vi "UDPsender.vi"() -> ()   [LabVIEW 2012]
panel:
  in  "Relative Time Step":u32
  in  "Time Reset":bool
  in  "Harvest Mode":bool[](array[boolean])
  in  "Throttle Mode":u16
  in  "Test Modes":bool[](array[boolean])
  in  "Channel Test Mode Config":bool[](array[boolean])
  in  "Sync Test Mode Config":bool[](array[boolean])
  in  "Sync Select":bool[](array[boolean])
  in  "Profiles Per Histogram":u16
  in  "Number of Bins":u16
  in  "User Reset":bool
  in  "Counts Per Bin":u16
  in  "Reset Profile Accumulator":bool[](array[boolean])
  in  "Channel Enable":bool[](array[boolean])
  in  "Sync Enable":bool[](array[boolean])
  in  "Reset":bool
  in  "Send":bool
  in  "Send Command, manual entry":string
  out "Sender Error":errorcluster
  in  "End Sender Program":bool
  # "valid range (2-4096)"
  # "valid range (2-4096)"
  # "valid range (1-32,768)"
  # "stop sender"
  # "valid range (0-7)"
  # "valid range (0-33,554,432)"
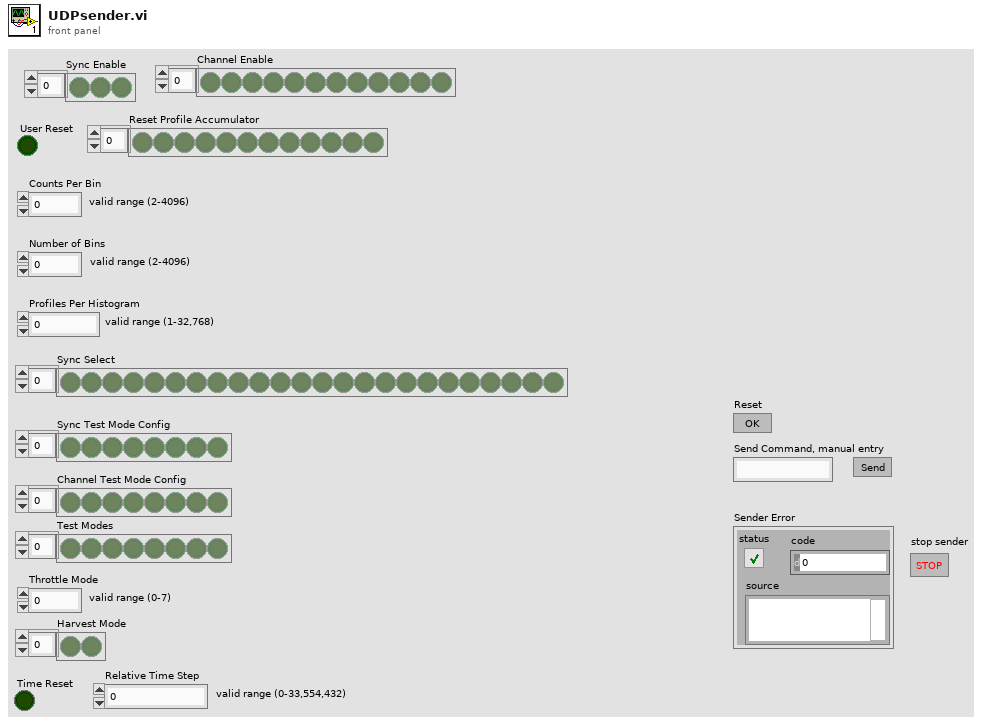
[diagram p1: front panel]
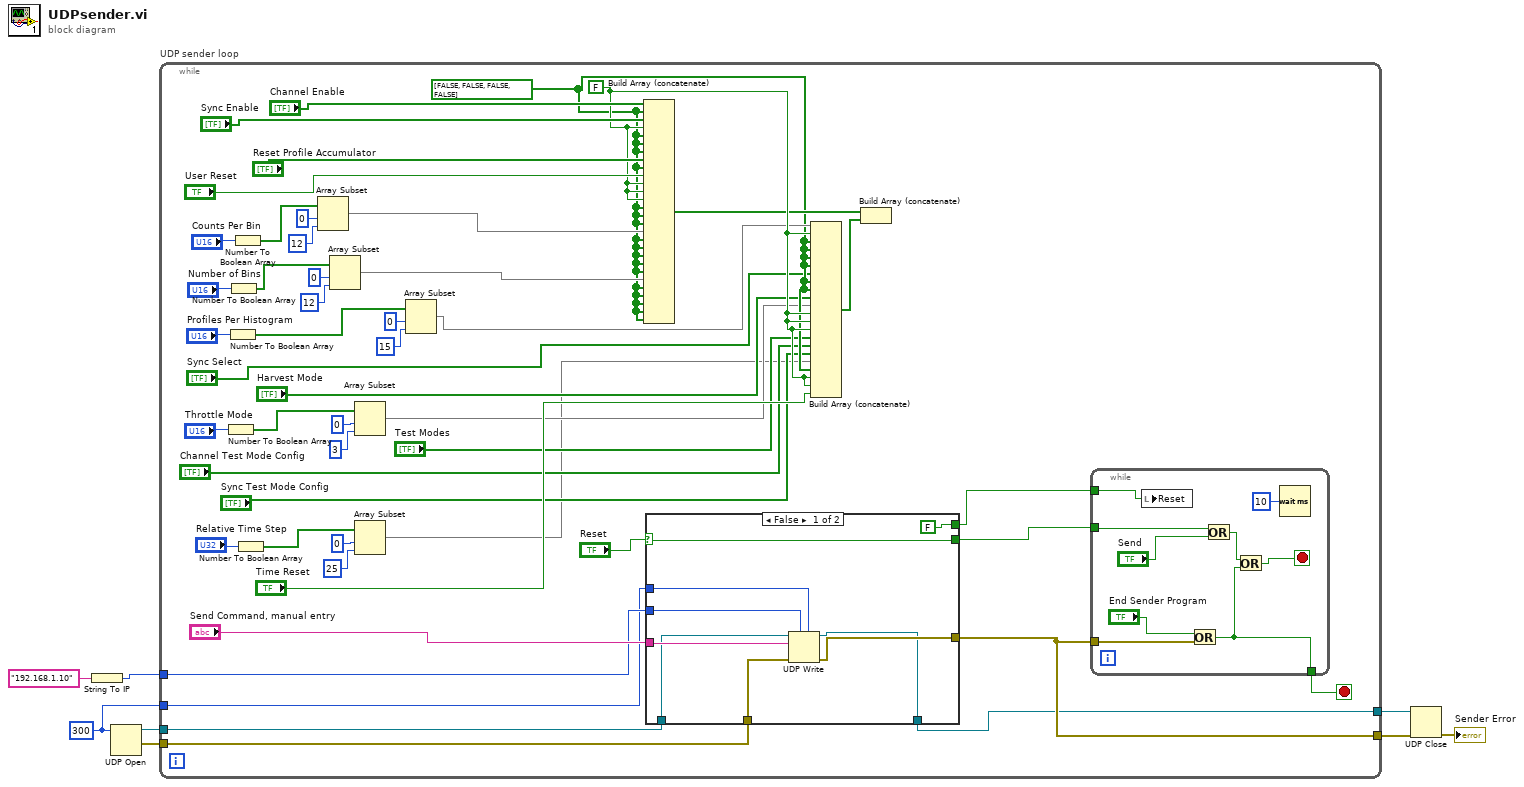
[diagram p0: block diagram]
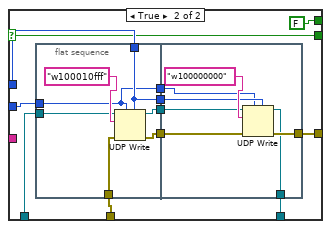
[diagram p2: hidden frame]
diagram:
  w1 = u16 300 ("port")
  n1 = String To IP(1:"192.168.1.10" ("name")) -> (0:w3:u32)
  n2 = UDP Open(11:w1) -> (port=w7:refnum<k16>, 0:w8:errorcluster)  [unwired: 4 in, 1 out]
  n3 = while "UDP sender loop" {
    tunnel: w8 -> [w55]
    tunnel: w7 -> [w53]
    tunnel: [w54] -> w6
    tunnel: w3 -> [w52]
    tunnel: [w25] -> w2
    tunnel: w1 -> [w50]
    stop <- w58 stop-if-true
    w16 = bool[] [FALSE, FALSE, FALSE, FALSE] ("appended array")
    w21 = FALSE ("Reset")
    n4 = Number To Boolean Array(number="Throttle Mode") -> (Boolean array=w26:bool[])
    n5 = Number To Boolean Array(number="Profiles Per Histogram") -> (Boolean array=w34:bool[])
    n6 = Number To Boolean Array(number="Number of Bins") -> (Boolean array=w37:bool[])
    n7 = Number To Boolean Array(number="Counts Per Bin") -> (Boolean array=w40:bool[])
    n8 = Number To Boolean Array(number="Relative Time Step") -> (Boolean array=w22:bool[])
    n9 = Array Subset(array=w40, index=0, length=12) -> (w30:bool[])
    n10 = Array Subset(array=w37, index=0, length=12) -> (w29:bool[])
    n11 = Array Subset(array=w26, index=0, length=3) -> (w13:bool[])
    n12 = Array Subset(array=w22, index=0, length=25) -> (w9:bool[])
    n13 = Array Subset(array=w34, index=0, length=15) -> (w17:bool[])
    n14 = Build Array (concatenate)("Channel Enable", w16, "Sync Enable", w21, w16, w16, w16, "Reset Profile Accumulator", w16, "User Reset", w21, w21, w21, w16, w16, w16, w30, w16, w16, w16, w16, w16, w29, w16, w16, w16, w16, w16) -> (w19:bool[])
    n15 = case shown="False" "Reset" {
      selector: "Reset" -> [w59 w68]
      tunnel: "Send Command, manual entry" -> [w67 _]
      tunnel: w55 -> [w65 w79]
      tunnel: [w64 w77] -> w54
      tunnel: w53 -> [w66 w74]
      tunnel: w50 -> [w61 w73]
      tunnel: w52 -> [w62 w71]
      tunnel: [FALSE ("Reset") FALSE ("Reset")] -> w49
      tunnel: [w59 w68] -> w51
      tunnel: [w63 w76] -> w25
      frame False {
        n16 = UDP Write(address=w62, port or service name=w61, connection ID=w66, data in=w67, 8:w65) -> (error out=w64:errorcluster, 3:w63:refnum<k16>)  [unwired: 1 in]
      }
      frame True {
        n17 = flat-sequence {
          tunnel: w79 -> [w85]
          tunnel: [w84] -> w78
          tunnel: [w83] -> w75
          tunnel: w74 -> [w82]
          tunnel: w73 -> [w81]
          tunnel: [w81] -> w72
          tunnel: w71 -> [w80]
          tunnel: [w80] -> w70
          tunnel: w78 -> [w92]
          tunnel: [w91] -> w77
          tunnel: [w90] -> w76
          tunnel: w75 -> [w89]
          tunnel: w72 -> [w88]
          tunnel: w70 -> [w87]
          frame #0 {
            n18 = UDP Write(address=w80, port or service name=w81, connection ID=w82, data in="w100010fff" ("F-format string"), 8:w85) -> (error out=w84:errorcluster, 3:w83:refnum<k16>)  [unwired: 1 in]
          }
          frame #1 {
            n19 = UDP Write(address=w87, port or service name=w88, connection ID=w89, data in="w100000000" ("F-format string"), 8:w92) -> (error out=w91:errorcluster, 3:w90:refnum<k16>)  [unwired: 1 in]
          }
        }
      }
    }
    n20 = Build Array (concatenate)(w17, w21, w16, w16, w16, w16, "Sync Select", w16, w16, "Harvest Mode", w13, w21, w21, w21, "Test Modes", "Channel Test Mode Config", "Sync Test Mode Config", w9, w16, w21, w21, "Time Reset") -> (w18:bool[])
    n21 = Build Array (concatenate)(w19, w18) -> ()  [unwired: 1 out]
    n22 = while {
      tunnel: w54 -> [w100]
      tunnel: [w98] -> w58
      tunnel: w51 -> [w97]
      tunnel: w49 -> [w94]
      stop <- w101 stop-if-true
      n23 = local write "Reset"(w94) -> ()
      n24 = Or(x="End Sender Program", y=w100) -> (x .or. y?=w98:bool)
      n25 = Or(x=w97, y="Send") -> (x .or. y?=w95:bool)
      n26 = Or(x=w95, y=w98) -> (x .or. y?=w101:bool)
      n27 = Wait (ms)(milliseconds to wait=u32 10) -> ()  [unwired: 1 out]
    }
  }
  n28 = UDP Close(connection ID=w2, 8:w6) -> (error out=→"Sender Error":errorcluster)  [unwired: 1 out]
